vi "USRP_singlecarrierTDMUSRP3_eve.vi"() -> ()   [LabVIEW 2021]
uses:
  <vilib>/addons/Modulation/Analog/controls/Complex Data Waveform.ctl
  <vilib>/Analysis/coordinate.llb/Angle Units.ctl
  <vilib>/Analysis/coordinate.llb/Angle Range (Degree).ctl
  <vilib>/Analysis/coordinate.llb/Wrap Angle (scalar).vi
  system stop.vi
  <vilib>/measure/matone.llb/Extract Single Tone Information 1 Chan (CDB).vi
  <instrlib>/niUSRP/niUSRP Fetch Rx Data (CDB Cluster).vi
  <vilib>/addons/Modulation/niAMT.lvlib
  <vilib>/measure/NI_MAPro.lvlib
  <vilib>/Analysis/NI_AAL_Angle.lvlib
panel:
  in  "Tab Control":T1(tab)
  in  "IQ rate":dbl=400000.0 format="%#_6p"
  in  "Rx IP":refnum<k15>="192.168.10.200"
  in  "Rx gain":dbl format="%#_6f"
  out "coerced IQ rate Rx":dbl=400000.0 format="%#_6p"
  out "coerced carrier frequency Rx":dbl=2400000000.0 format="%#_6p"
  in  "number of samples":i64=4000
  in  "carrier frequency":dbl=2400000000.0 format="%#_6p"
  out "PilotUSRP1":bool
  out "PilotUSRP2":bool
  out "detected frequency":dbl=9960.325350983943 format="%.2p"
  out "Rx Waveform":dbl[](graph)
  out "detected Amplitude in dBm":dbl format="%.2p"
  out "detected Amplitude in dBm 2":dbl format="%.2p"
  out "detected frequency 2":dbl=9960.325350983943 format="%.2p"
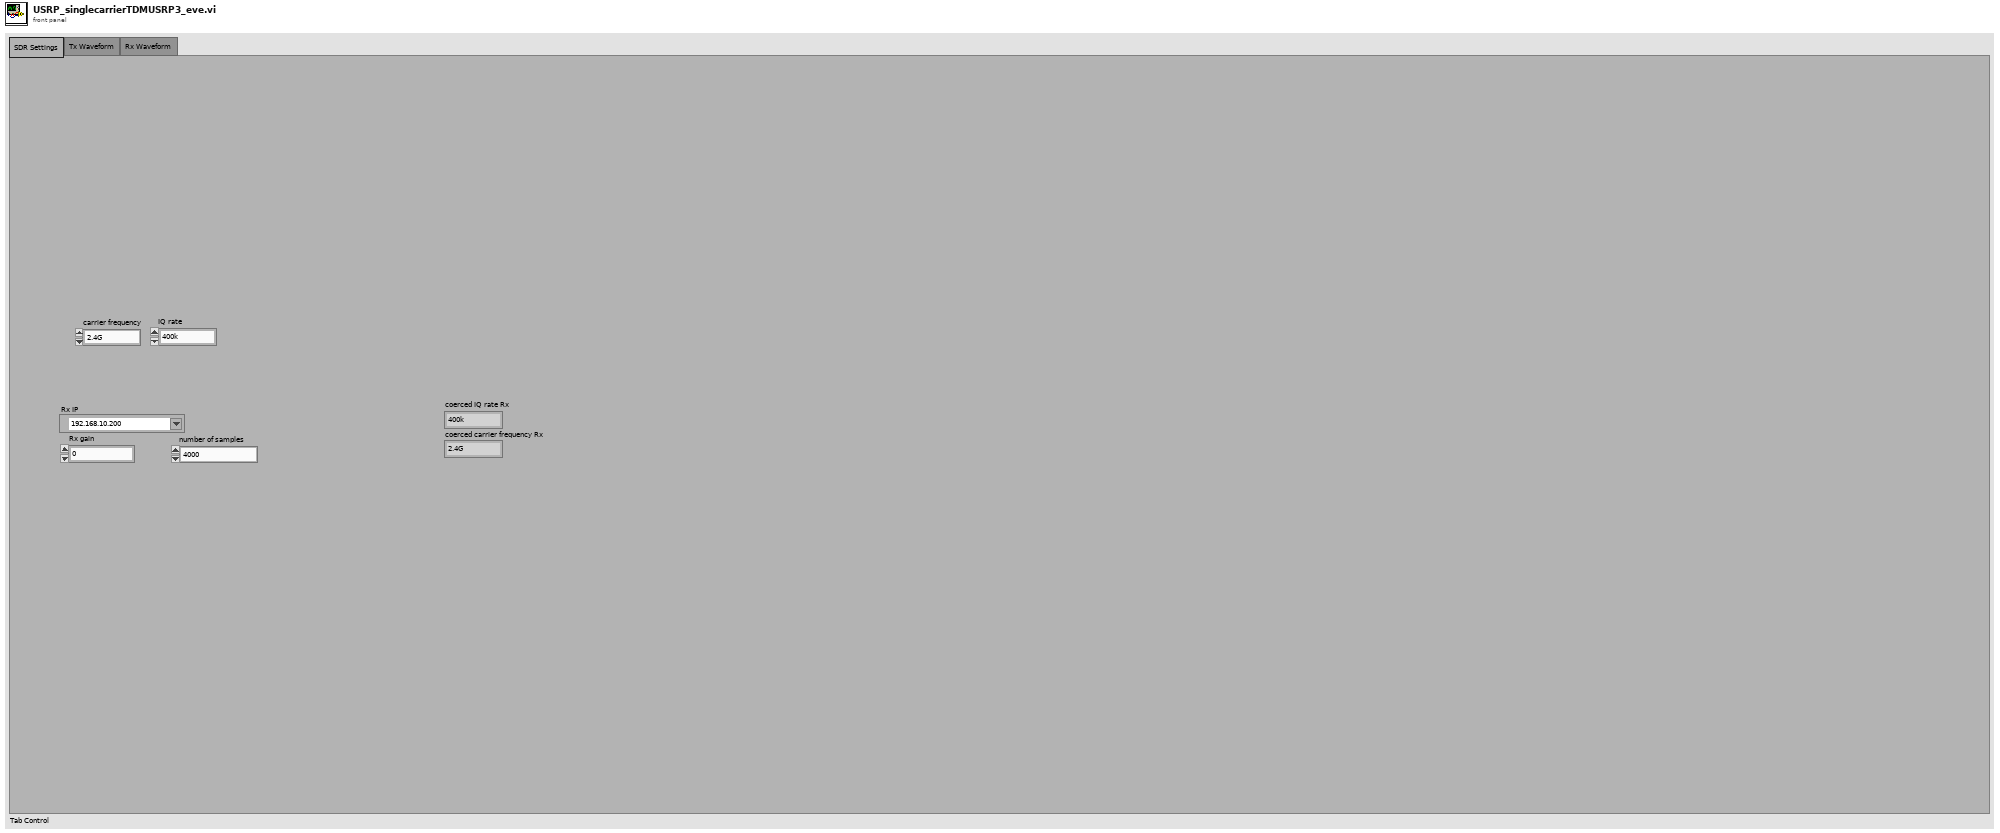
[diagram p1: front panel]
types:
  T1 = enum32{"SDR Settings", "Tx Waveform", "Rx Waveform"}
  T2 = typedef "niAMT.lvlib/Complex Data Waveform.ctl" = cluster{"t0":dbl, "dt":dbl, "Y":cdb[]}
  T3 = typedef "NI_AAL_Angle.lvlib/Angle Range (Degree).ctl" = u16
  T4 = typedef "NI_AAL_Angle.lvlib/Angle Units.ctl" = i32
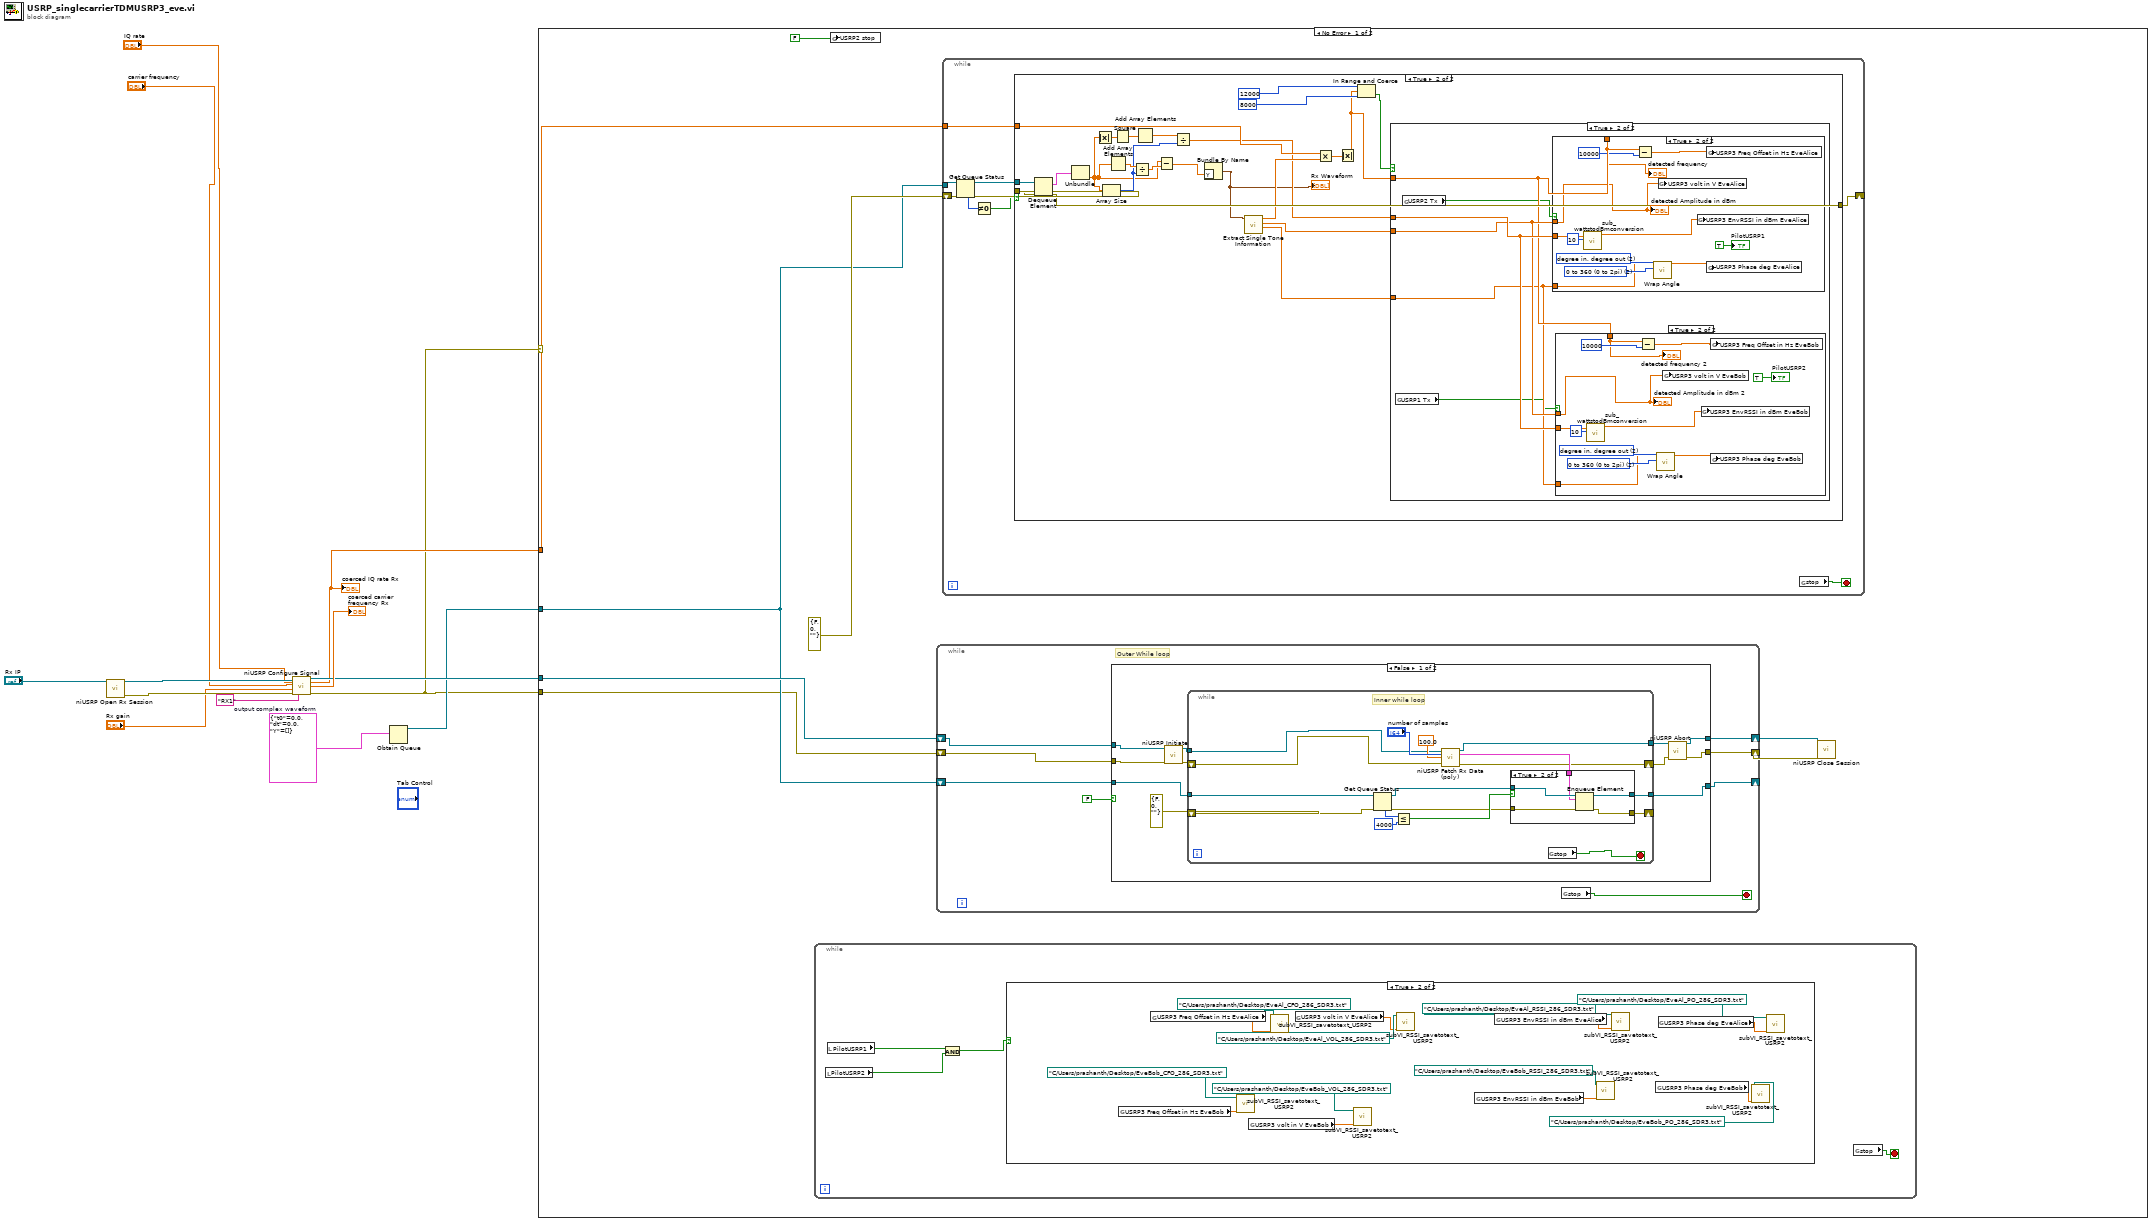
[diagram p0: block diagram]
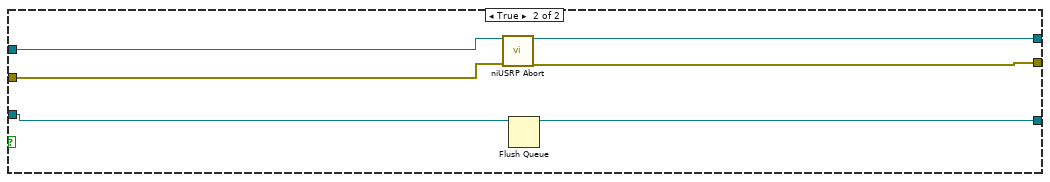
[diagram p4: hidden frame]
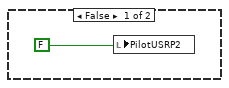
[diagram p7: hidden frame]
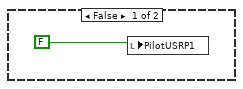
[diagram p8: hidden frame]
diagram:
  w6 = T2 {"t0"=0.0, "dt"=0.0, "Y"=[]}  # output complex waveform
  n1 = call <instrlib>:"niUSRP Open Rx Session.vi"("device names"="Rx IP") -> ("session handle out"=w12:refnum<k15>, "error out"=w11:errorcluster)  [unwired: 13 in]
  n2 = call <instrlib>:"niUSRP Configure Signal.vi"("session handle"=w12, "IQ rate"="IQ rate", "carrier frequency"="carrier frequency", "gain"="Rx gain", "error in (no error)"=w11, "active antenna"="RX1") -> ("session handle out"=w7:refnum<k15>, "coerced IQ rate"=w4:dbl, "coerced carrier frequency"=→"coerced carrier frequency Rx":dbl, "error out"=w1:errorcluster)  [unwired: 5 in, 1 out]
  "coerced IQ rate Rx" <- w4
  n3 = Obtain Queue(element data type=w6) -> (queue out=w5:refnum<queue>)  [unwired: 4 in, 2 out]
  n4 = case shown="No Error" w1 {
    tunnel: w7 -> [w20 _]
    tunnel: w5 -> [w19 _]
    tunnel: w4 -> [w18 _]
    tunnel: w1 -> [w17 _]
    frame No Error {
      n5 = while {
        stop <- w25 stop-if-true
        n6 = local read "PilotUSRP2"() -> (w23:bool)
        n7 = local read "PilotUSRP1"() -> (w24:bool)
        n8 = And(x=w24, y=w23) -> (x .and. y?=w22:bool)
        n9 = case shown="True" w22 {
          frame False {
          }
          frame True {
            n10 = global read "system stop.vi" "USRP3 Freq Offset in Hz EveBob"() -> (w37:dbl)
            n11 = global read "system stop.vi" "USRP3 Freq Offset in Hz EveAlice"() -> (w40:dbl)
            n12 = call "subVI_RSSI_savetotext_USRP2.vi"("RSSI"=w37, "file path (dialog if empty)"=path "C:/Users/prashanth/Desktop/EveBob_CFO_286_SDR3.txt") -> ()  [unwired: 10 in]
            n13 = global read "system stop.vi" "USRP3 volt in V EveBob"() -> (w35:dbl)
            n14 = call "subVI_RSSI_savetotext_USRP2.vi"("RSSI"=w40, "file path (dialog if empty)"=path "C:/Users/prashanth/Desktop/EveAl_CFO_286_SDR3.txt") -> ()  [unwired: 10 in]
            n15 = global read "system stop.vi" "USRP3 volt in V EveAlice"() -> (w38:dbl)
            n16 = call "subVI_RSSI_savetotext_USRP2.vi"("RSSI"=w35, "file path (dialog if empty)"=path "C:/Users/prashanth/Desktop/EveBob_VOL_286_SDR3.txt") -> ()  [unwired: 10 in]
            n17 = call "subVI_RSSI_savetotext_USRP2.vi"("RSSI"=w38, "file path (dialog if empty)"=path "C:/Users/prashanth/Desktop/EveAl_VOL_286_SDR3.txt") -> ()  [unwired: 10 in]
            n18 = global read "system stop.vi" "USRP3 EnvRSSI in dBm EveBob"() -> (w32:dbl)
            n19 = global read "system stop.vi" "USRP3 EnvRSSI in dBm EveAlice"() -> (w34:dbl)
            n20 = call "subVI_RSSI_savetotext_USRP2.vi"("RSSI"=w32, "file path (dialog if empty)"=path "C:/Users/prashanth/Desktop/EveBob_RSSI_286_SDR3.txt") -> ()  [unwired: 10 in]
            n21 = call "subVI_RSSI_savetotext_USRP2.vi"("RSSI"=w34, "file path (dialog if empty)"=path "C:/Users/prashanth/Desktop/EveAl_RSSI_286_SDR3.txt") -> ()  [unwired: 10 in]
            n22 = global read "system stop.vi" "USRP3 Phase deg EveBob"() -> (w27:dbl)
            n23 = global read "system stop.vi" "USRP3 Phase deg EveAlice"() -> (w30:dbl)
            n24 = call "subVI_RSSI_savetotext_USRP2.vi"("RSSI"=w27, "file path (dialog if empty)"=path "C:/Users/prashanth/Desktop/EveBob_PO_286_SDR3.txt") -> ()  [unwired: 10 in]
            n25 = call "subVI_RSSI_savetotext_USRP2.vi"("RSSI"=w30, "file path (dialog if empty)"=path "C:/Users/prashanth/Desktop/EveAl_PO_286_SDR3.txt") -> ()  [unwired: 10 in]
          }
        }
        n26 = global read "system stop.vi" "stop"() -> (w25:bool)
      }
      n27 = global write "system stop.vi" "USRP2 stop"(FALSE) -> ()
      n28 = while {
        shift-right: [w48] -> w15
        shift-left: w20 -> [w45]
        shift-right: [w47] -> w14
        shift-left: w17 -> [w46]
        shift-right: [w44] -> _
        shift-left: w19 -> [w49]
        stop <- w42 stop-if-true
        # "Outer While loop"
        n29 = case shown="False" FALSE {
          tunnel: w49 -> [w60 w88]
          tunnel: [w55 w90] -> w48
          tunnel: [w54 w89] -> w47
          tunnel: w46 -> [w51 w86]
          tunnel: w45 -> [w52 w87]
          tunnel: [w50 w85] -> w44
          frame False {
            n30 = call <instrlib>:"niUSRP Initiate.vi"("session handle"=w52, "error in (no error)"=w51) -> ("session handle out"=w58:refnum<k15>, "error out"=w57:errorcluster)  [unwired: 12 in]
            n31 = while {
              tunnel: w60 -> [w77]
              shift-right: [w65] -> w53
              shift-left: w57 -> [w63]
              shift-right: [w76] -> _
              shift-left: errorcluster {"status"=FALSE, "code"=0, "source"=""} ("error in (no error)") -> [w75]
              tunnel: w58 -> [w64]
              tunnel: [w66] -> w56
              tunnel: [w62] -> w50
              stop <- w61 stop-if-true
              # "Inner while loop"
              n32 = Get Queue Status(queue=w77, error in (no error)=w75) -> (queue out=w70:refnum<queue>, error out=w71:errorcluster, # elements in queue=w74:i32)  [unwired: 1 in, 5 out]
              n33 = Less Or Equal?(x=w74, y=4000) -> (x <= y?=w72:bool)
              n34 = call-poly <instrlib>:"niUSRP Fetch Rx Data (poly).vi"("session handle"=w64, "number of samples"="number of samples", "timeout"=100.0, "error in (no error)"=w63) -> ("session handle out"=w66:refnum<k15>, "data"=w68:cluster{"t0":dbl, "dt":dbl, "Y":cdb[]}, "error out"=w65:errorcluster)  [unwired: 8 in, 1 out]
              n35 = case shown="True" w72 {
                tunnel: w71 -> [w79 w84]
                tunnel: w70 -> [w78 w83]
                tunnel: w68 -> [_ w82]
                tunnel: [w79 w81] -> w76
                tunnel: [w78 w80] -> w62
                frame False {
                }
                frame True {
                  n36 = Enqueue Element(queue=w83, element=w82, error in (no error)=w84) -> (queue out=w80:refnum<queue>, error out=w81:errorcluster)  [unwired: 1 in, 1 out]
                }
              }
              n37 = global read "system stop.vi" "stop"() -> (w61:bool)
            }
            n38 = call <instrlib>:"niUSRP Abort.vi"("session handle"=w56, "error in (no error)"=w53) -> ("session handle out"=w55:refnum<k15>, "error out"=w54:errorcluster)  [unwired: 12 in]
          }
          frame True {
            n39 = call <instrlib>:"niUSRP Abort.vi"("session handle"=w87, "error in (no error)"=w86) -> ("session handle out"=w90:refnum<k15>, "error out"=w89:errorcluster)  [unwired: 12 in]
            n40 = Flush Queue(queue=w88) -> (queue out=w85:refnum<queue>)  [unwired: 1 in, 2 out]
          }
        }
        n41 = global read "system stop.vi" "stop"() -> (w42:bool)
      }
      n42 = while {
        tunnel: w19 -> [w96]
        shift-right: [w91] -> _
        shift-left: errorcluster {"status"=FALSE, "code"=0, "source"=""} ("error in (no error)") -> [w95]
        tunnel: w18 -> [w93]
        stop <- w92 stop-if-true
        n43 = Get Queue Status(queue=w96, error in (no error)=w95) -> (queue out=w98:refnum<queue>, error out=w97:errorcluster, # elements in queue=w99:i32)  [unwired: 1 in, 5 out]
        n44 = Not Equal To 0?(x=w99) -> (x != 0?=w94:bool)
        n45 = case shown="True" w94 {
          tunnel: w98 -> [_ w123]
          tunnel: w97 -> [w100 w122]
          tunnel: [w100 w120] -> w91
          tunnel: w93 -> [_ w113]
          frame False {
          }
          frame True {
            n46 = Dequeue Element(queue=w123, error in (no error)=w122) -> (element=w121:T2, error out=w120:errorcluster)  [unwired: 1 in, 2 out]
            n47 = Unbundle(w121) -> ("Y"=w105:cdb[])  [unwired: 2 out]
            n48 = Absolute Value(x=w105) -> (abs(x)=w110:dbl[])
            n49 = Array Size(array=w105) -> (size(s)=w107:i32)
            n50 = Add Array Elements(numeric array=w105) -> (sum=w119:cdb)
            n51 = Square(x=w110) -> (x^2=w109:dbl[])
            n52 = Divide(x=w119, y=w107) -> (x/y=w118:cdb)
            n53 = Add Array Elements(numeric array=w109) -> (sum=w108:dbl)
            n54 = Subtract(x=w105, y=w118) -> (x-y=w117:cdb[])
            n55 = Divide(x=w108, y=w107) -> (x/y=w106:dbl)
            n56 = Bundle By Name("Y"=w117) -> (w104:waveform(cdb))  [unwired: 1 in]
            "Rx Waveform" <- w104
            n57 = call-poly <vilib>:"Extract Single Tone Information.vi"("time signal in"=w104) -> ("detected phase (deg)"=w102:dbl, "detected amplitude"=w103:dbl, "detected frequency"=w114:dbl)  [unwired: 5 in, 3 out]
            n58 = Multiply(x=w113, y=w114) -> (x*y=w112:dbl)
            n59 = Absolute Value(x=w112) -> (abs(x)=w111:dbl)
            n60 = In Range and Coerce(upper limit=12000, x=w111, lower limit=8000) -> (In Range?=w101:bool)  [unwired: 1 out]
            n61 = case shown="True" w101 {
              tunnel: w111 -> [_ w127]
              tunnel: w106 -> [_ w129]
              tunnel: w103 -> [_ w128]
              tunnel: w102 -> [_ w126]
              frame False {
              }
              frame True {
                n62 = global read "system stop.vi" "USRP1 Tx"() -> (w125:bool)
                n63 = global read "system stop.vi" "USRP2 Tx"() -> (w124:bool)
                n64 = case shown="True" w124 {
                  tunnel: w128 -> [_ w148]
                  tunnel: w129 -> [_ w147]
                  tunnel: w127 -> [_ w146]
                  tunnel: w126 -> [_ w145]
                  frame False {
                    n65 = local write "PilotUSRP1"(FALSE) -> ()
                  }
                  frame True {
                    w151 = T3 2 items=["none", "-180 to 180 (-pi to pi)", "0 to 360 (0 to 2pi)"] ("angle range")
                    w152 = T4 2 items=["radian in, radian out", "radian in, degree out", "degree in, degree out", "degree in, radian out"] ("angle units")
                    n66 = call "sub_wattstodBmconversion.vi"("Amp or Power"=10, "detected amplitude"=w147) -> ("Numeric"=w153:dbl)  [unwired: 9 in]
                    n67 = Subtract(x=w146, y=10000) -> (x-y=w154:dbl)
                    n68 = call-poly <vilib>:"Wrap Angle.vi"("angle units"=w152, "angle range"=w151, "angle in"=w145) -> ("angle out"=w150:dbl)  [unwired: 7 in, 1 out]
                    n69 = global write "system stop.vi" "USRP3 volt in V EveAlice"(w148) -> ()
                    n70 = global write "system stop.vi" "USRP3 EnvRSSI in dBm EveAlice"(w153) -> ()
                    n71 = global write "system stop.vi" "USRP3 Freq Offset in Hz EveAlice"(w154) -> ()
                    n72 = global write "system stop.vi" "USRP3 Phase deg EveAlice"(w150) -> ()
                    "detected frequency" <- w146
                    "detected Amplitude in dBm" <- w148
                    "PilotUSRP1" <- TRUE
                  }
                }
                n73 = case shown="True" w125 {
                  tunnel: w128 -> [_ w135]
                  tunnel: w129 -> [_ w134]
                  tunnel: w127 -> [_ w133]
                  tunnel: w126 -> [_ w132]
                  frame False {
                    n74 = local write "PilotUSRP2"(FALSE) -> ()
                  }
                  frame True {
                    w138 = T3 2 items=["none", "-180 to 180 (-pi to pi)", "0 to 360 (0 to 2pi)"] ("angle range")
                    w139 = T4 2 items=["radian in, radian out", "radian in, degree out", "degree in, degree out", "degree in, radian out"] ("angle units")
                    n75 = call "sub_wattstodBmconversion.vi"("Amp or Power"=10, "detected amplitude"=w134) -> ("Numeric"=w140:dbl)  [unwired: 9 in]
                    n76 = Subtract(x=w133, y=10000) -> (x-y=w141:dbl)
                    n77 = call-poly <vilib>:"Wrap Angle.vi"("angle units"=w139, "angle range"=w138, "angle in"=w132) -> ("angle out"=w137:dbl)  [unwired: 7 in, 1 out]
                    n78 = global write "system stop.vi" "USRP3 volt in V EveBob"(w135) -> ()
                    n79 = global write "system stop.vi" "USRP3 EnvRSSI in dBm EveBob"(w140) -> ()
                    n80 = global write "system stop.vi" "USRP3 Freq Offset in Hz EveBob"(w141) -> ()
                    n81 = global write "system stop.vi" "USRP3 Phase deg EveBob"(w137) -> ()
                    "detected frequency 2" <- w133
                    "detected Amplitude in dBm 2" <- w135
                    "PilotUSRP2" <- TRUE
                  }
                }
              }
            }
          }
        }
        n82 = global read "system stop.vi" "stop"() -> (w92:bool)
      }
      n83 = call <instrlib>:"niUSRP Close Session.vi"("session handle"=w15, "error in (no error)"=w14) -> ()  [unwired: 13 in, 1 out]
    }
    frame Error {
    }
  }
